vi "AddViToProject.vi"(5 "PropertyFolderName":string, 7 "Property":string, 8 "error out 2":errorcluster, 9 "PropertyNode":bool, 10 "NewVIPath":path, 11 "ProjectFolder":refnum<vi>) -> (0 "error out":errorcluster, 3 "AddFile":refnum<vi>)   [LabVIEW 2012, in "ClassWriterNative.lvclass"]
uses:
  <resource>/Framework/Providers/Open_GDS/ClassProviders/Provider_LvNativeClass/ClassWriterNative_class/ClassWriterNative.lvclass
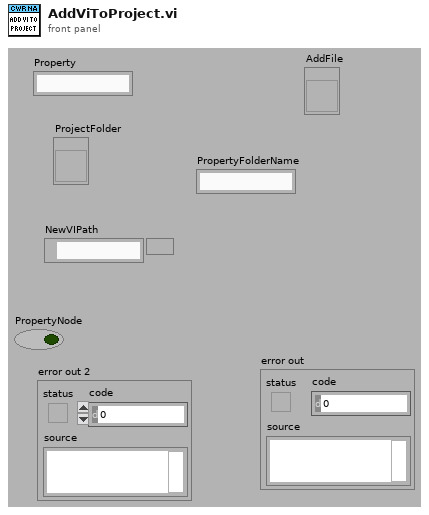
[diagram p1: front panel]
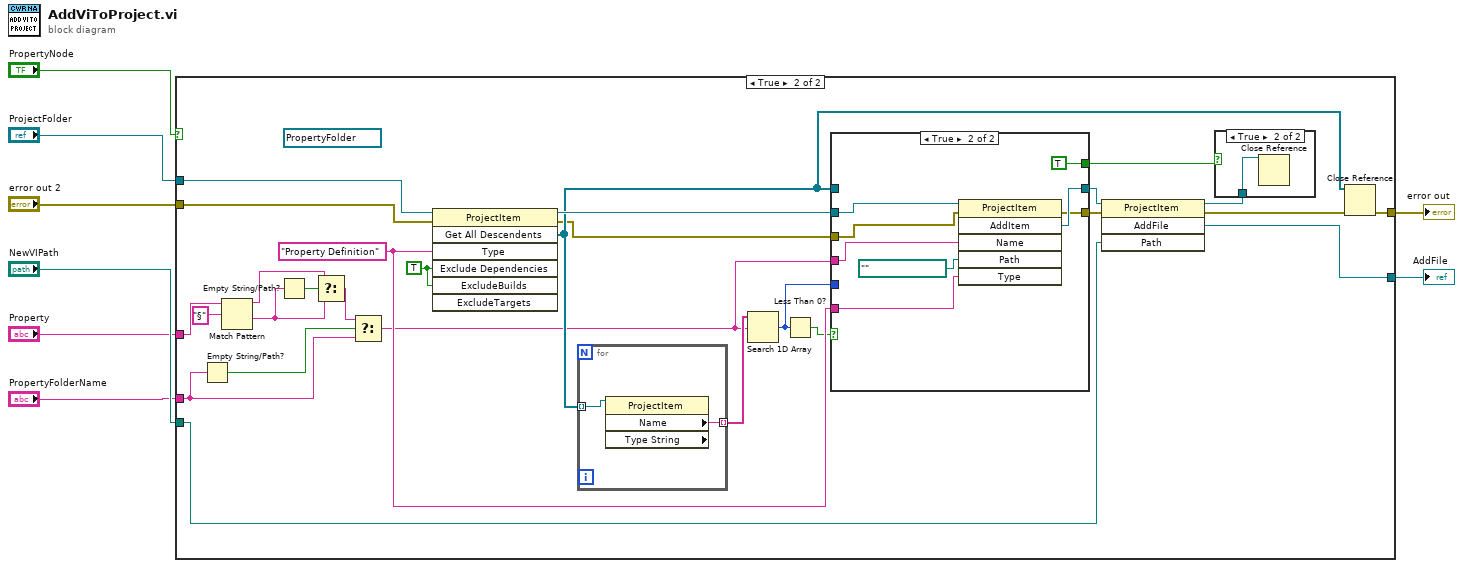
[diagram p0: block diagram]
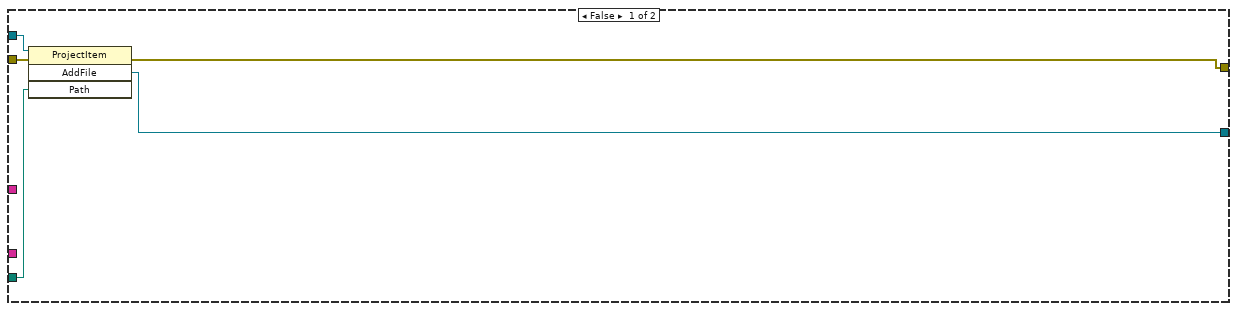
[diagram p2: hidden frame]
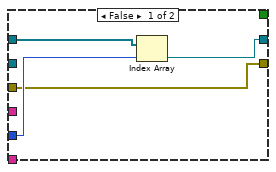
[diagram p4: hidden frame]
diagram:
  n1 = case shown="True" "PropertyNode" {
    tunnel: "ProjectFolder" -> [w13 w38]
    tunnel: "NewVIPath" -> [w12 w32]
    tunnel: "error out 2" -> [w11 w39]
    tunnel: [w10 w31] -> w7
    tunnel: [w9 w25] -> w1
    tunnel: "Property" -> [_ w27]
    tunnel: "PropertyFolderName" -> [_ w23]
    frame False {
      n2 = invoke class="ProjectItem" method="AddFile"(reference=w13, error in=w11, "Path"=w12) -> (error out=w9:errorcluster, "AddFile"=w10:refnum<vi>)  [unwired: 1 in, 2 out]
    }
    frame True {
      (unwired) refnum<vi> refnum ("reference out")
      w40 = TRUE ("ExcludeDependencies")
      w35 = "Property Definition" ("Type")
      n3 = Empty String/Path?(string/path=w23) -> (empty?=w24:bool)
      n4 = Match Pattern(string=w27, regular expression="§") -> (before substring=w17:string, after substring=w14:string)  [unwired: 1 in, 2 out]
      n5 = Empty String/Path?(string/path=w14) -> (empty?=w16:bool)
      n6 = Select(t=w17, s=w16, f=w14) -> (s? t:f=w15:string)
      n7 = Select(t=w15, s=w24, f=w23) -> (s? t:f=w22:string)
      n8 = invoke class="ProjectItem" method="Get All Descendents"(reference=w38, error in=w39, "Type"=w35, "Exclude Dependencies"=w40, "ExcludeBuilds"=w40) -> (reference out=w36:refnum<vi>, error out=w20:errorcluster, "All Descendents"=w29:refnum<vi>[])  [unwired: 2 in, 4 out]
      n9 = for {
        tunnel: w29 -> [w55] mode=indexing
        tunnel: [w54] -> w37 mode=indexing
        n10 = property class="ProjectItem" props=["Name", "Type String"](reference=w55) -> ("Name"=w54:string)  [unwired: 1 in, 3 out]
      }
      n11 = Search 1D Array(1D array=w37, element=w22) -> (index of element=w21:i32)  [unwired: 1 in]
      n12 = Less Than 0?(x=w21) -> (x < 0?=w26:bool)
      n13 = case shown="True" w26 {
        tunnel: w36 -> [_ w53]
        tunnel: w22 -> [_ w52]
        tunnel: w35 -> [_ w50]
        tunnel: [w44 w49] -> w34
        tunnel: [w42 w48] -> w33
        tunnel: w29 -> [w45 _]
        tunnel: w21 -> [w43 _]
        tunnel: w20 -> [w42 w47]
        tunnel: [_ TRUE] -> w19
        frame False {
          n14 = Index Array(array=w45, index=w43) -> (element=w44:refnum<vi>)
        }
        frame True {
          n15 = invoke class="ProjectItem" method="AddItem"(reference=w53, error in=w47, "Name"=w52, "Path"=path "", "Type"=w50) -> (error out=w48:errorcluster, "AddItem"=w49:refnum<vi>)  [unwired: 1 in, 4 out]
        }
      }
      n16 = invoke class="ProjectItem" method="AddFile"(reference=w34, error in=w33, "Path"=w32) -> (reference out=w18:refnum<vi>, error out=w30:errorcluster, "AddFile"=w31:refnum<vi>)  [unwired: 1 in, 1 out]
      n17 = case shown="True" w19 {
        tunnel: w18 -> [_ w41]
        frame False {
        }
        frame True {
          n18 = Close Reference(reference=w41) -> ()  [unwired: 1 in, 1 out]
        }
      }
      n19 = Close Reference(reference=w29, error in (no error)=w30) -> (error out=w25:errorcluster)
    }
  }
  "error out" <- w1
  "AddFile" <- w7
